vi "excel数据到bool的转化4x4.vi"() -> ()   [LabVIEW 2018]
uses:
  <vilib>/Utility/NIReport.llb/Report Type.ctl
  <vilib>/addons/_office/excel.llb/Excel Get Data ([dbl]).vi
  <vilib>/Utility/NIReport.llb/NI_report.lvclass
  <vilib>/addons/_office/NI_ReportGenerationToolkit.lvlib
  <vilib>/Utility/NIReport.llb/NI_ReportGenerationCore.lvlib
  <vilib>/Utility/NIReport.llb/Excel/NI_Excel.lvclass
panel:
  out "x-y":u32
  out "all":T1
  out "32x1":T2
  out "初始化的数组":bool[](array[boolean])
  out "输出数组":dbl[](array[numeric])
  in  "end (-1, -1)":cluster{"row":i32, "column":i32}={"row"=-1, "column"=-1}
  in  "start (-1, -1)":cluster{"row":i32, "column":i32}={"row"=-1, "column"=-1}
  out "data":dbl[][](array[numeric]) format="%.5f"
  out "error out":errorcluster caption="错误输出"
  in  "template (empty)":path caption="模板（空）"
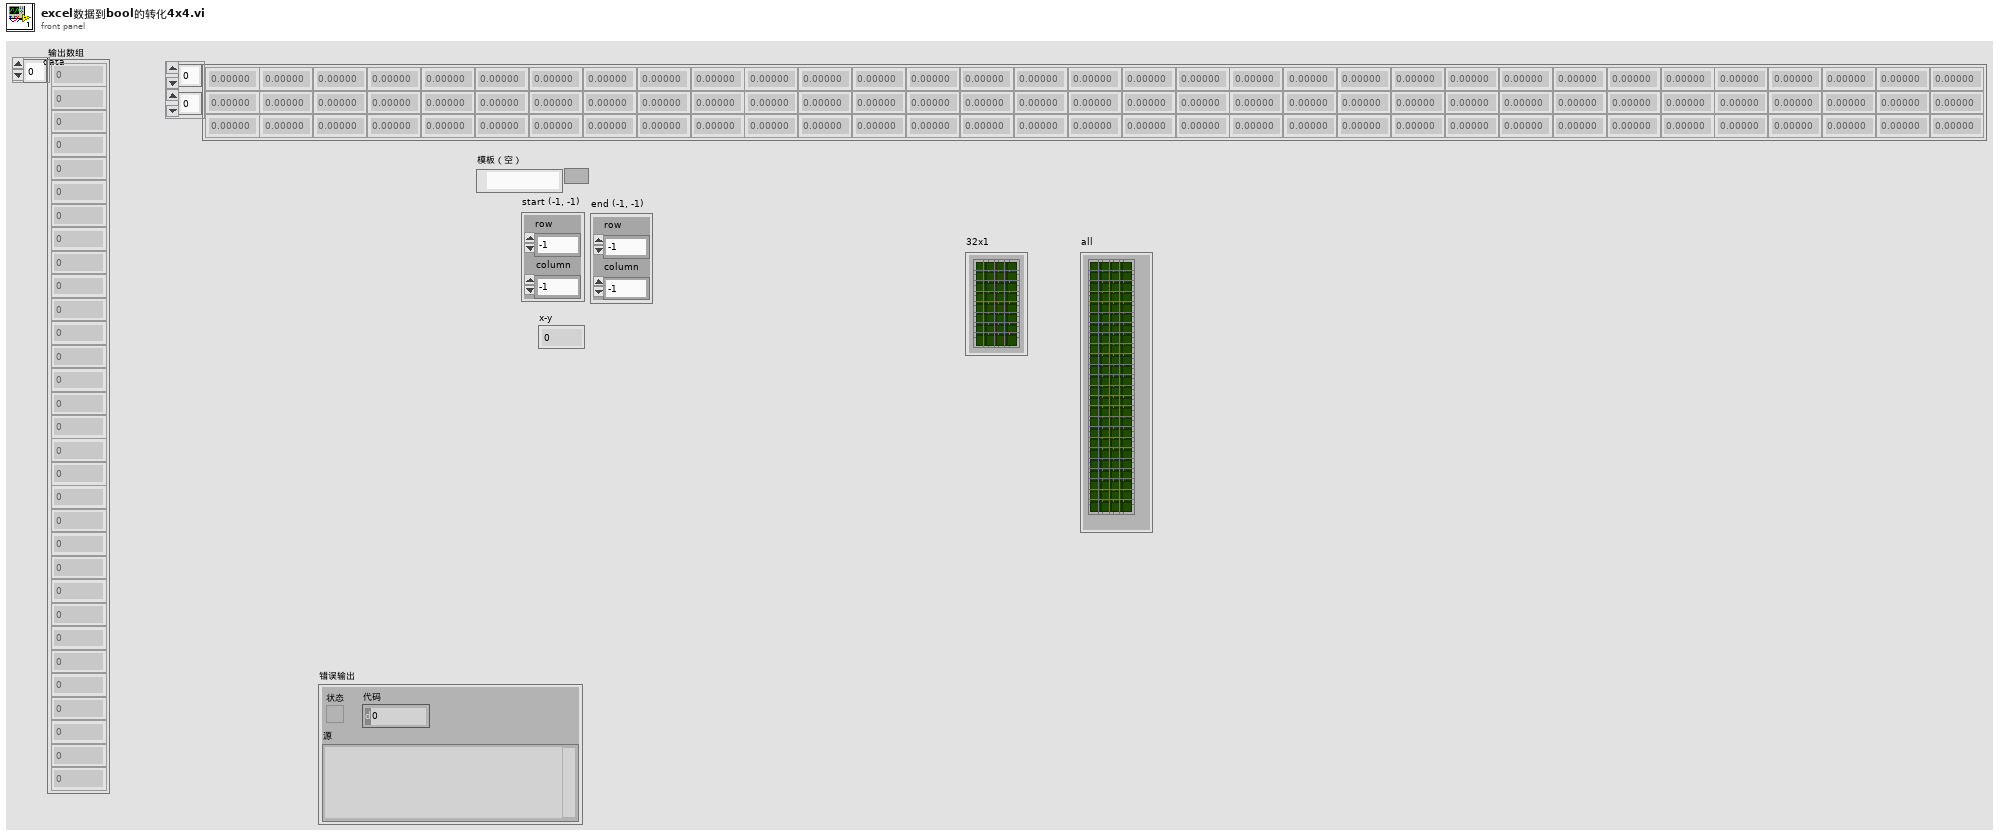
[diagram p1: front panel]
types:
  T1 = cluster{"布尔":bool, "布尔 2":bool, "布尔 3":bool, "布尔 4":bool, "布尔 5":bool, "布尔 6":bool, "布尔 7":bool, "布尔 8":bool, "布尔 9":bool, "布尔 10":bool, "布尔 11":bool, "布尔 12":bool, "布尔 13":bool, "布尔 14":bool, "布尔 15":bool, "布尔 16":bool, "布尔 17":bool, "布尔 18":bool, "布尔 19":bool, "布尔 20":bool, "布尔 21":bool, "布尔 22":bool, "布尔 23":bool, "布尔 24":bool, "布尔 25":bool, "布尔 26":bool, "布尔 27":bool, "布尔 28":bool, "布尔 29":bool, "布尔 30":bool, "布尔 31":bool, "布尔 32":bool, "布尔 33":bool, "布尔 34":bool, "布尔 35":bool, "布尔 36":bool, "布尔 37":bool, "布尔 38":bool, "布尔 39":bool, "布尔 40":bool, "布尔 41":bool, "布尔 42":bool, "布尔 43":bool, "布尔 44":bool, "布尔 45":bool, "布尔 46":bool, "布尔 47":bool, "布尔 48":bool, "布尔 49":bool, "布尔 50":bool, "布尔 51":bool, "布尔 52":bool, "布尔 53":bool, "布尔 54":bool, "布尔 55":bool, "布尔 56":bool, "布尔 57":bool, "布尔 58":bool, "布尔 59":bool, "布尔 60":bool, "布尔 61":bool, "布尔 62":bool, "布尔 63":bool, "布尔 64":bool, "布尔 65":bool, "布尔 66":bool, "布尔 67":bool, "布尔 68":bool, "布尔 69":bool, "布尔 70":bool, "布尔 71":bool, "布尔 72":bool, "布尔 73":bool, "布尔 74":bool, "布尔 75":bool, "布尔 76":bool, "布尔 77":bool, "布尔 78":bool, "布尔 79":bool, "布尔 80":bool, "布尔 81":bool, "布尔 82":bool, "布尔 83":bool, "布尔 84":bool, "布尔 85":bool, "布尔 86":bool, "布尔 87":bool, "布尔 88":bool, "布尔 89":bool, "布尔 90":bool, "布尔 91":bool, "布尔 92":bool, "布尔 93":bool, "布尔 94":bool, "布尔 95":bool, "布尔 96":bool}
  T2 = cluster{"布尔":bool, "布尔 2":bool, "布尔 3":bool, "布尔 4":bool, "布尔 5":bool, "布尔 6":bool, "布尔 7":bool, "布尔 8":bool, "布尔 9":bool, "布尔 10":bool, "布尔 11":bool, "布尔 12":bool, "布尔 13":bool, "布尔 14":bool, "布尔 15":bool, "布尔 16":bool, "布尔 17":bool, "布尔 18":bool, "布尔 19":bool, "布尔 20":bool, "布尔 21":bool, "布尔 22":bool, "布尔 23":bool, "布尔 24":bool, "布尔 25":bool, "布尔 26":bool, "布尔 27":bool, "布尔 28":bool, "布尔 29":bool, "布尔 30":bool, "布尔 31":bool, "布尔 32":bool}
  T3 = typedef "NI_ReportGenerationCore.lvlib/Report Type.ctl" = enum16{"HTML", "Word", "Excel"}
  T4 = enum16{"maximized", "minimized", "normal", "no change"}
  T5 = cluster{"[0]":bool, "[1]":bool, "[2]":bool, "[3]":bool, "[4]":bool, "[5]":bool, "[6]":bool, "[7]":bool, "[8]":bool, "[9]":bool, "[10]":bool, "[11]":bool, "[12]":bool, "[13]":bool, "[14]":bool, "[15]":bool, "[16]":bool, "[17]":bool, "[18]":bool, "[19]":bool, "[20]":bool, "[21]":bool, "[22]":bool, "[23]":bool, "[24]":bool, "[25]":bool, "[26]":bool, "[27]":bool, "[28]":bool, "[29]":bool, "[30]":bool, "[31]":bool}
  T6 = cluster{"初始化的数组[0]":bool, "初始化的数组[1]":bool, "初始化的数组[2]":bool, "初始化的数组[3]":bool, "初始化的数组[4]":bool, "初始化的数组[5]":bool, "初始化的数组[6]":bool, "初始化的数组[7]":bool, "初始化的数组[8]":bool, "初始化的数组[9]":bool, "初始化的数组[10]":bool, "初始化的数组[11]":bool, "初始化的数组[12]":bool, "初始化的数组[13]":bool, "初始化的数组[14]":bool, "初始化的数组[15]":bool, "初始化的数组[16]":bool, "初始化的数组[17]":bool, "初始化的数组[18]":bool, "初始化的数组[19]":bool, "初始化的数组[20]":bool, "初始化的数组[21]":bool, "初始化的数组[22]":bool, "初始化的数组[23]":bool, "初始化的数组[24]":bool, "初始化的数组[25]":bool, "初始化的数组[26]":bool, "初始化的数组[27]":bool, "初始化的数组[28]":bool, "初始化的数组[29]":bool, "初始化的数组[30]":bool, "初始化的数组[31]":bool, "初始化的数组[32]":bool, "初始化的数组[33]":bool, "初始化的数组[34]":bool, "初始化的数组[35]":bool, "初始化的数组[36]":bool, "初始化的数组[37]":bool, "初始化的数组[38]":bool, "初始化的数组[39]":bool, "初始化的数组[40]":bool, "初始化的数组[41]":bool, "初始化的数组[42]":bool, "初始化的数组[43]":bool, "初始化的数组[44]":bool, "初始化的数组[45]":bool, "初始化的数组[46]":bool, "初始化的数组[47]":bool, "初始化的数组[48]":bool, "初始化的数组[49]":bool, "初始化的数组[50]":bool, "初始化的数组[51]":bool, "初始化的数组[52]":bool, "初始化的数组[53]":bool, "初始化的数组[54]":bool, "初始化的数组[55]":bool, "初始化的数组[56]":bool, "初始化的数组[57]":bool, "初始化的数组[58]":bool, "初始化的数组[59]":bool, "初始化的数组[60]":bool, "初始化的数组[61]":bool, "初始化的数组[62]":bool, "初始化的数组[63]":bool, "初始化的数组[64]":bool, "初始化的数组[65]":bool, "初始化的数组[66]":bool, "初始化的数组[67]":bool, "初始化的数组[68]":bool, "初始化的数组[69]":bool, "初始化的数组[70]":bool, "初始化的数组[71]":bool, "初始化的数组[72]":bool, "初始化的数组[73]":bool, "初始化的数组[74]":bool, "初始化的数组[75]":bool, "初始化的数组[76]":bool, "初始化的数组[77]":bool, "初始化的数组[78]":bool, "初始化的数组[79]":bool, "初始化的数组[80]":bool, "初始化的数组[81]":bool, "初始化的数组[82]":bool, "初始化的数组[83]":bool, "初始化的数组[84]":bool, "初始化的数组[85]":bool, "初始化的数组[86]":bool, "初始化的数组[87]":bool, "初始化的数组[88]":bool, "初始化的数组[89]":bool, "初始化的数组[90]":bool, "初始化的数组[91]":bool, "初始化的数组[92]":bool, "初始化的数组[93]":bool, "初始化的数组[94]":bool, "初始化的数组[95]":bool}
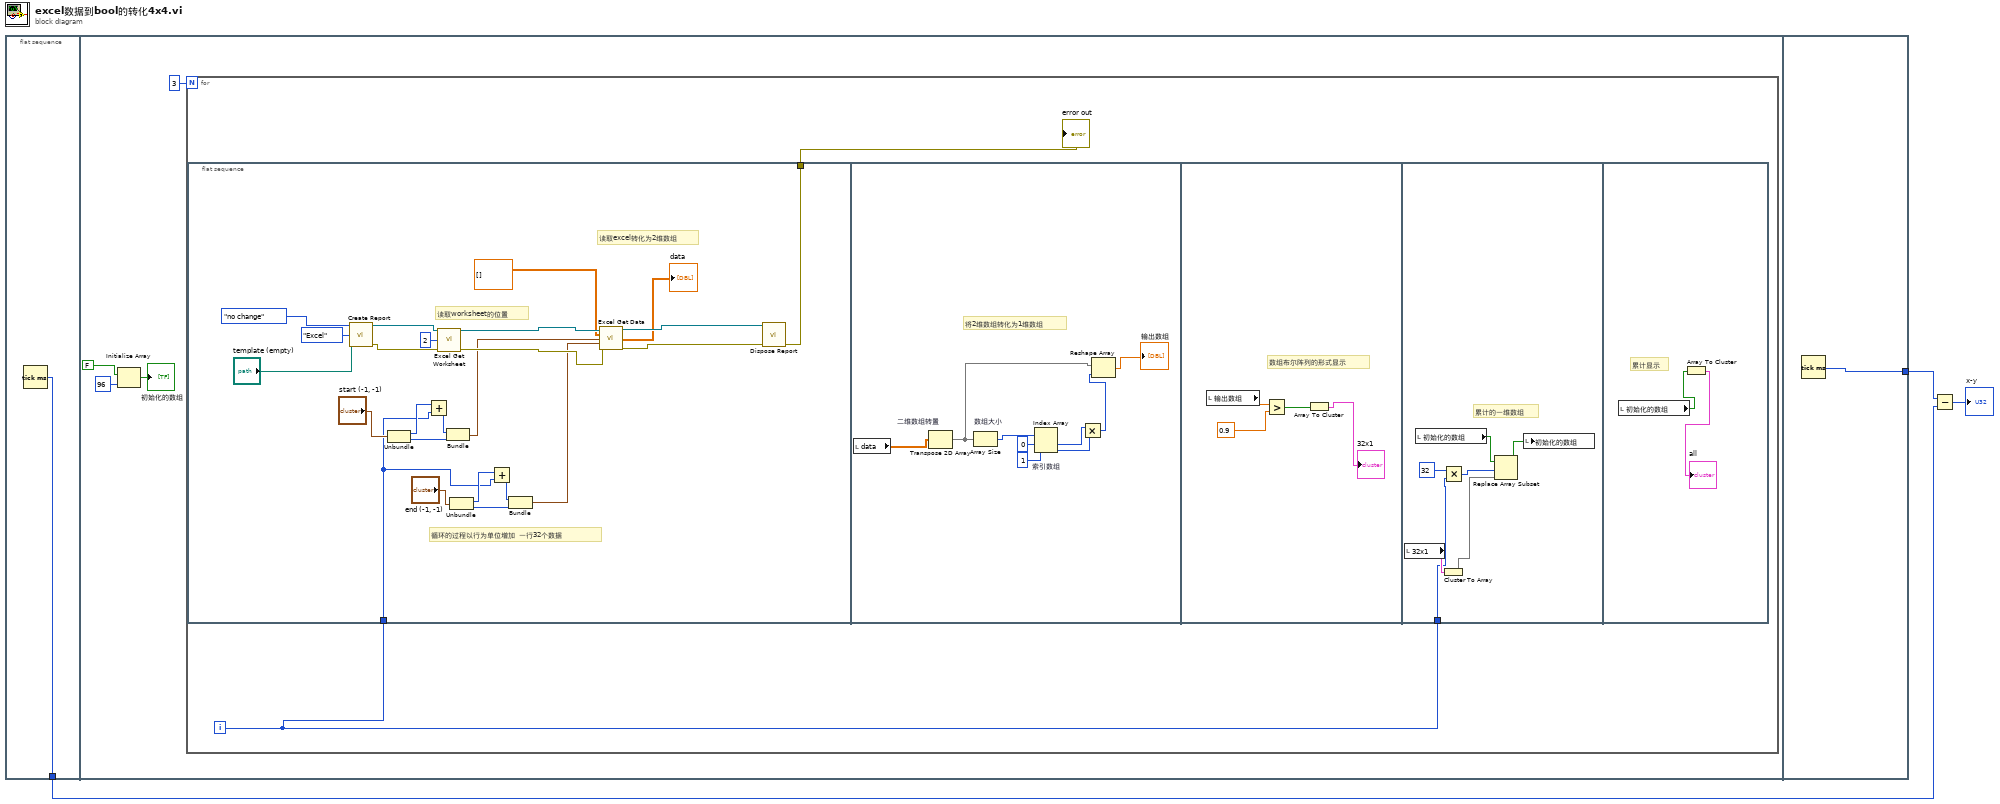
[diagram p0: block diagram]
diagram:
  n1 = flat-sequence {
    tunnel: [w4] -> w2
    tunnel: [w57] -> w3
    frame #0 {
      n2 = Tick Count (ms)() -> (millisecond timer value=w4:u32)
    }
    frame #1 {
      n3 = Initialize Array(FALSE, 96 ("维数大小")) -> (→"初始化的数组":bool[])
      n4 = for {
        N: 3 -> [_]
        i -> [w9]
        n5 = flat-sequence {
          tunnel: [w22] -> w10
          tunnel: w9 -> [w12]
          tunnel: w9 -> [w49]
          frame #0 {
            # "循环的过程以行为单位增加  一行32个数据"
            # "读取worksheet的位置"
            # "读取excel转化为2维数组"
            n6 = call <vilib>:"Create Report.vi"("window state (normal)"=T4."no change", "report type"=Report_Type."Excel", "template (empty)"="template (empty)") -> ("report out"=w31:refnum<class "NI_report.lvclass">, "error out"=w30:errorcluster)  [unwired: 11 in]
            n7 = Unbundle("start (-1, -1)") -> ("row"=w19:i32, "column"=w20:i32)
            n8 = Add(x=w19, y=w12) -> (x+y=w18:i32)
            n9 = call <vilib>:"Excel Get Worksheet.vi"("report in"=w31, "worksheet index (0)"=2, "error in (no error)"=w30) -> ("report out"=w28:refnum<class "NI_report.lvclass">, "error out"=w27:errorcluster)  [unwired: 11 in]
            n10 = Bundle(w18, "column"=w20) -> (w17:cluster{i32, "column":i32})  [unwired: 1 in]
            n11 = Unbundle("end (-1, -1)") -> ("row"=w15:i32, "column"=w14:i32)
            n12 = Add(x=w15, y=w12) -> (x+y=w16:i32)
            n13 = Bundle(w16, "column"=w14) -> (w11:cluster{i32, "column":i32})  [unwired: 1 in]
            n14 = call-poly <vilib>:"Excel Get Data.vi"("report in"=w28, "data type"=dbl[][] [], "start (-1, -1)"=w17, "end (-1, -1)"=w11, "error in (no error)"=w27) -> ("report out"=w26:refnum<class "NI_report.lvclass">, "data"=→"data":dbl[][], "error out"=w25:errorcluster)  [unwired: 8 in]
            n15 = call-dynamic "Dispose Report.vi"("report in"=w26, "error in (no error)"=w25) -> ("error out"=w22:errorcluster)  [unwired: 13 in]
          }
          frame #1 {
            # "将2维数组转化为1维数组"
            n16 = local read "data"() -> (w38:dbl[][])
            n17 = Transpose 2D Array "二维数组转置"(2D array=w38) -> (transposed array=w39:dbl[][])
            n18 = Array Size "数组大小"(array=w39) -> (size(s)=w40:i32[])
            n19 = Index Array "索引数组"(array=w40, index #1=0 ("索引"), index #2=1 ("索引")) -> (element #1=w41:i32, element #2=w42:i32)
            n20 = Multiply(x=w41, y=w42) -> (x*y=w43:i32)
            n21 = Reshape Array(w39, w43) -> (→"输出数组":dbl[])
          }
          frame #2 {
            # "数组布尔阵列的形式显示"
            n22 = local read "输出数组"() -> (w46:dbl[])
            n23 = Greater?(x=w46, y=0.9) -> (0:w47:bool[])
            n24 = Array To Cluster(array=w47) -> (cluster=→"32x1":T5)
          }
          frame #3 {
            # "累计的一维数组"
            n25 = local read "32x1"() -> (w50:T2)
            n26 = local read "初始化的数组"() -> (w53:bool[])
            n27 = Cluster To Array(cluster=w50) -> (array=w52:bool[])
            n28 = Multiply(x=32, y=w49) -> (x*y=w51:i32)
            n29 = Replace Array Subset(array=w53, new element=w52, index=w51) -> (w54:bool[])
            n30 = local write "初始化的数组"(w54) -> ()
          }
          frame #4 {
            # "累计显示"
            n31 = local read "初始化的数组"() -> (w56:bool[])
            n32 = Array To Cluster(array=w56) -> (cluster=→"all":T6)
          }
        }
        "error out" <- w10
      }
    }
    frame #2 {
      n33 = Tick Count (ms)() -> (millisecond timer value=w57:u32)
    }
  }
  n34 = Subtract(x=w3, y=w2) -> (x-y=→"x-y":u32)
